vi "get best scope range.vi"(1 "Set point":dbl, 2 "Range Strings and Values":T1) -> (0 "Best Range":dbl(ring)=700.0 items=["200V"=200.0, "700V"=700.0, "1400V"=1400.0])   [LabVIEW 2018]
uses:
  <vilib>/Utility/miscctls.llb/LVStringsAndValuesArrayTypeDef_DBL.ctl
panel:
  # "Get the best scope voltage or current range for the a given NHR set point"
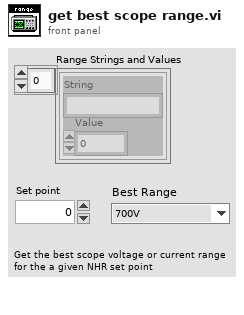
[diagram p1: front panel]
types:
  T1 = typedef "LVStringsAndValuesArrayTypeDef_DBL.ctl" = cluster{"String":string, "Value":dbl}[]
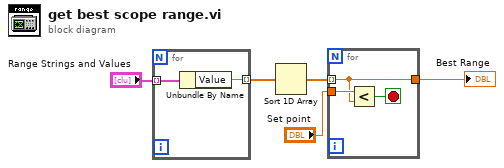
[diagram p0: block diagram]
diagram:
  n1 = for {
    tunnel: "Range Strings and Values" -> [w7] mode=indexing
    tunnel: [w6] -> w5 mode=indexing
    n2 = Unbundle By Name(w7) -> ("Value"=w6:dbl)
  }
  n3 = Sort 1D Array(array=w5) -> (sorted array=w4:dbl[])
  n4 = for {
    tunnel: w4 -> [w8] mode=indexing
    tunnel: "Set point" -> [w9]
    tunnel: [w8] -> w2
    stop <- w10 stop-if-true
    n5 = Less?(x=w9, y=w8) -> (x < y?=w10:bool)
  }
  "Best Range" <- w2
